vi "Upload to S3.vi"(8 "error in (no error)":errorcluster, 11 "Control Experiment in":refnum<class "Control Experiment SM.lvclass">) -> (0 "error out":errorcluster, 3 "Control Experiment out":refnum<class "Control Experiment SM.lvclass">)   [LabVIEW 2016, in "Control Experiment SM.lvclass"]
uses:
  Control Experiment SM.lvclass
  Control Experiment SM.lvclass/Control Experiment SM.ctl
  <userlib>/LevyLab/postgreSQL-timescaleDB/Data.S3/Data.S3.lvclass
panel:
  out "Object Path":string
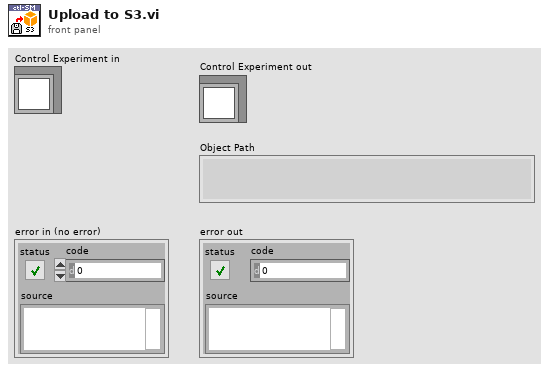
[diagram p1: front panel]
types:
  T1 = typedef "Control Experiment SM.lvclass/Instrument--enum.ctl" = enum16{"----- AFM/EBL -----", "AGILENT", "CYPHER", "Gemini2", "JEOL", "MFP3D", "----- Cryostat -----", "CF900", "DR200", "MNK", "PPMS 1", "PPMS 2", "PPMS 3", "----- Optics -----", "THz 1", "THz 2"}
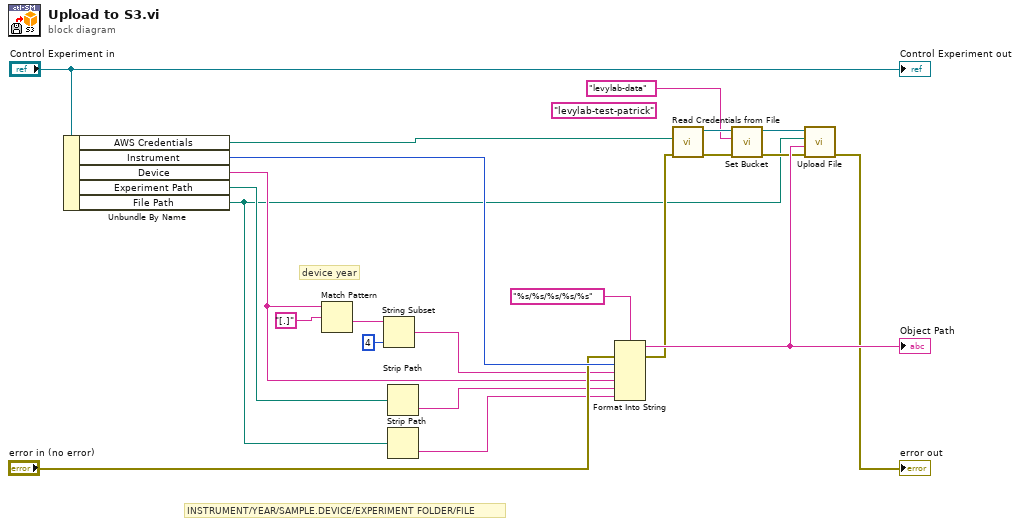
[diagram p0: block diagram]
diagram:
  (unwired) "levylab-test-patrick" ("Bucket name")
  # "INSTRUMENT/YEAR/SAMPLE.DEVICE/EXPERIMENT FOLDER/FILE"
  # "device year"
  n1 = Unbundle By Name("Control Experiment in") -> ("AWS Credentials"=w15:path, "Instrument"=w17:T1, "Device"=w9:string, "Experiment Path"=w16:path, "File Path"=w1:path)
  n2 = Match Pattern(string=w9, regular expression="[.]" ("delimiter (Tab)")) -> (after substring=w18:string)  [unwired: 1 in, 3 out]
  n3 = String Subset(string=w18, length (rest)=4 ("length (rest)")) -> (substring=w10:string)  [unwired: 1 in]
  n4 = Strip Path(path=w16) -> (name=w8:string)  [unwired: 1 out]
  n5 = Strip Path(path=w1) -> (name=w7:string)  [unwired: 1 out]
  n6 = Format Into String(format string="%s/%s/%s/%s/%s", error in="error in (no error)", w17, w10, w9, w8, w7) -> (resulting string=w20:string, error out=w12:errorcluster)  [unwired: 1 in]
  "Object Path" <- w20
  n7 = call <userlib>:"Read Credentials from File.vi"("error in (no error)"=w12, "path to aws credentials"=w15) -> ("error out"=w6:errorcluster, "Data.S3 out"=w5:refnum<class "Data.S3.lvclass">)  [unwired: 8 in]
  n8 = call <userlib>:"Set Bucket.vi"("error in (no error)"=w6, "Bucket name"="levylab-data", "Data.S3"=w5) -> ("error out"=w3:errorcluster, "Data.S3"=w4:refnum<class "Data.S3.lvclass">)  [unwired: 7 in]
  n9 = call <userlib>:"Upload File.vi"("error in (no error)"=w3, "Object Path (including file name)"=w20, "file to upload"=w1, "Data.S3"=w4) -> ("error out"=→"error out":errorcluster)  [unwired: 6 in, 1 out]
  "Control Experiment out" <- "Control Experiment in"
